vi "Thruster control commnd algorithm with fwd and rev RHP.vi"(3 "RPM Measured":dbl=1.0, 4 "RPM Set":dbl=1.0 min=-1600.0 max=1600.0) -> (0 "Estimated Force":dbl=1.492471782203008 format="%#.3f", 1 "Control Voltage":dbl=1.492471782203008 format="%#.3f")   [LabVIEW 2021]
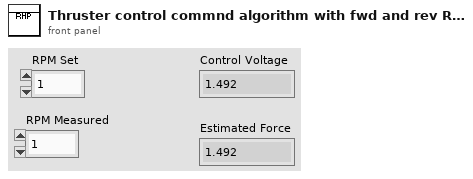
[diagram p1: front panel]
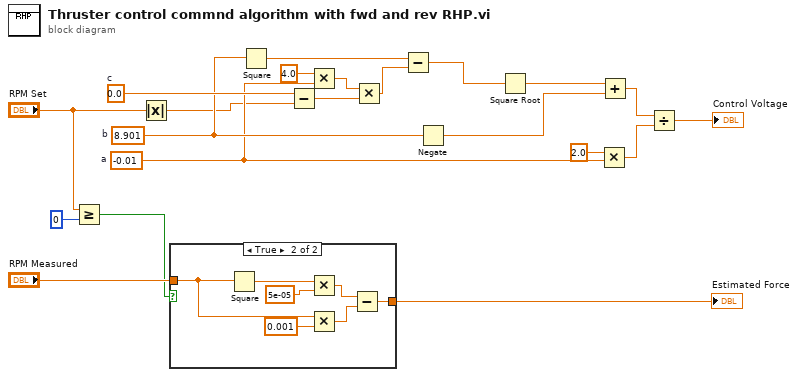
[diagram p0: block diagram]
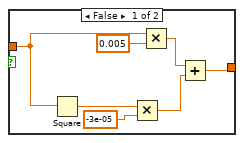
[diagram p2: hidden frame]
diagram:
  w21 = 0.0  # c
  w7 = -0.01  # a
  w20 = 8.901  # b
  n1 = Greater Or Equal?(x="RPM Set", y=i16 0) -> (x >= y?=w3:bool)
  n2 = Absolute Value(x="RPM Set") -> (abs(x)=w2:dbl)
  n3 = case shown="True" w3 {
    tunnel: [w22 w31] -> w6
    tunnel: "RPM Measured" -> [w23 w29]
    frame False {
      n4 = Square(x=w23) -> (x^2=w26:dbl)
      n5 = Multiply(x=w26, y=-3e-05) -> (x*y=w28:dbl)
      n6 = Multiply(x=w23, y=0.005) -> (x*y=w27:dbl)
      n7 = Add(x=w27, y=w28) -> (x+y=w22:dbl)
    }
    frame True {
      n8 = Square(x=w29) -> (x^2=w30:dbl)
      n9 = Multiply(x=w30, y=5e-05) -> (x*y=w34:dbl)
      n10 = Multiply(x=w29, y=0.001) -> (x*y=w33:dbl)
      n11 = Subtract(x=w34, y=w33) -> (x-y=w31:dbl)
    }
  }
  "Estimated Force" <- w6
  n12 = Square(x=w20) -> (x^2=w19:dbl)
  n13 = Subtract(x=w21, y=w2) -> (x-y=w10:dbl)
  n14 = Multiply(x=4.0, y=w7) -> (x*y=w16:dbl)
  n15 = Multiply(x=w16, y=w10) -> (x*y=w18:dbl)
  n16 = Subtract(x=w19, y=w18) -> (x-y=w15:dbl)
  n17 = Negate(x=w20) -> (-x=w13:dbl)
  n18 = Square Root(x=w15) -> (sqrt(x)=w14:dbl)
  n19 = Multiply(x=2.0, y=w7) -> (x*y=w11:dbl)
  n20 = Add(x=w14, y=w13) -> (x+y=w12:dbl)
  n21 = Divide(x=w12, y=w11) -> (x/y=→"Control Voltage":dbl)
